vi "getTestDataPath.vi"() -> (3 "testDataPath":path)   [LabVIEW 2018]
doc: "Get the test data path (vi files by ts_sal)."
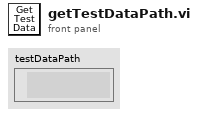
[diagram p1: front panel]
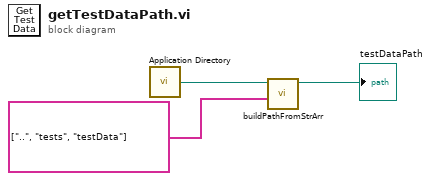
[diagram p0: block diagram]
diagram:
  n1 = call <vilib>:"Application Directory.vi"() -> ("Application Directory"=w2:path)
  n2 = call "buildPathFromStrArr.vi"("String Array"=string[] ["..", "tests", "testData"], "Root Path"=w2) -> ("Absolute Path"=→"testDataPath":path)  [unwired: 9 in]
